vi "3.5-Limbic.vi"() -> ()   [LabVIEW 2010]
uses:
  3.0-Global.vi
panel:
  out "size(s)":i32[](array[numeric])
  out "Waveform Graph":dbl[](graph)
  out "Drivable Paths":dbl[](array[numeric])
  out "Ogrid":u8[][](graph)
  out "Heartbeat":bool
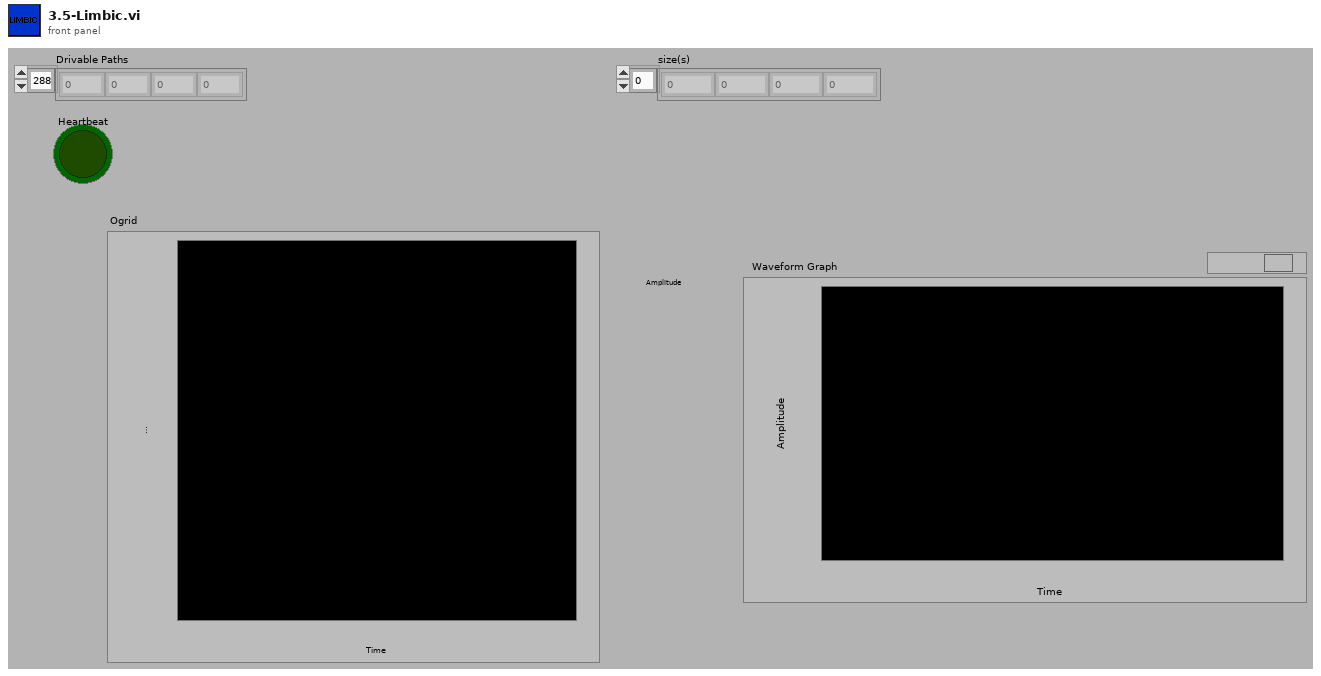
[diagram p1: front panel]
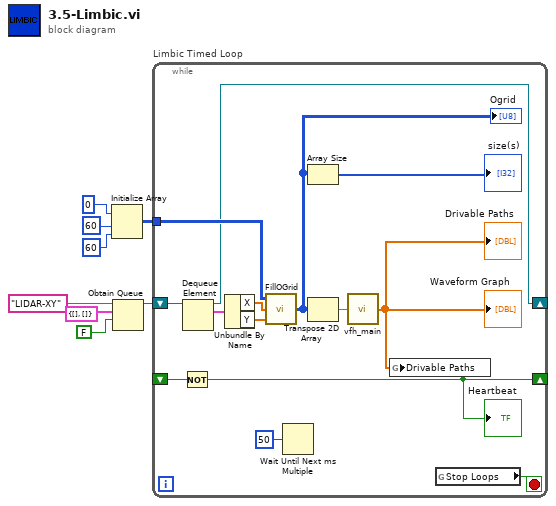
[diagram p0: block diagram]
diagram:
  n1 = Initialize Array(u8 0 ("element"), 60 ("dimension size"), 60 ("dimension size")) -> (w2:u8[][])
  n2 = Obtain Queue(name (unnamed)="LIDAR-XY", element data type=cluster{"X":dbl[], "Y":dbl[]} {"X"=[], "Y"=[]} ("output cluster"), create if not found? (T)=FALSE) -> (queue out=w1:refnum<queue>)  [unwired: 2 in, 2 out]
  n3 = while "Limbic Timed Loop" {
    shift-right: [w21] -> _
    shift-left: _ -> [w22]
    shift-right: [w19] -> _
    shift-left: w1 -> [w18]
    tunnel: w2 -> [w20]
    stop <- w10 stop-if-true
    n4 = Not(x=w22) -> (.not. x?=w21:bool)
    "Heartbeat" <- w21
    n5 = Dequeue Element(queue=w18) -> (queue out=w19:refnum<queue>, element=w17:cluster{"X":dbl[], "Y":dbl[]})  [unwired: 2 in, 2 out]
    n6 = Unbundle By Name(w17) -> ("X"=w16:dbl[], "Y"=w15:dbl[])
    n7 = call "FillOGrid.vi"("Y"=w15, "X"=w16, "OGrid In"=w20) -> ("OGrid Out"=w13:u8[][])
    "Ogrid" <- w13
    n8 = Wait Until Next ms Multiple(millisecond multiple=u32 50) -> ()  [unwired: 1 out]
    n9 = Array Size(array=w13) -> (size(s)=→"size(s)":i32[])
    n10 = Transpose 2D Array(2D array=w13) -> (transposed array=w12:u8[][])
    n11 = call "vfh_main.vi"("Local Occupancy Grid"=w12) -> ("Scaled Angles (-45 -> 45)"=w11:dbl[])
    "Drivable Paths" <- w11
    "Waveform Graph" <- w11
    n12 = global write "3.0-Global.vi" "Drivable Paths"(w11) -> ()
    n13 = global read "3.0-Global.vi" "Stop Loops"() -> (w10:bool)
  }
